vi "target.vi"   [LabVIEW 2020]
uses:
  <vilib>/rvi/interface/RandomDataEmulation/niFpgaRandomDataHandleErrors.vi
  <vilib>/rvi/DataTransferAndStorage/Container/XNode/niFpgaContainer.xnode
  <vilib>/rvi/interface/RandomDataEmulation/nirviRandomDataFpgaReadWriteTemplate.vi
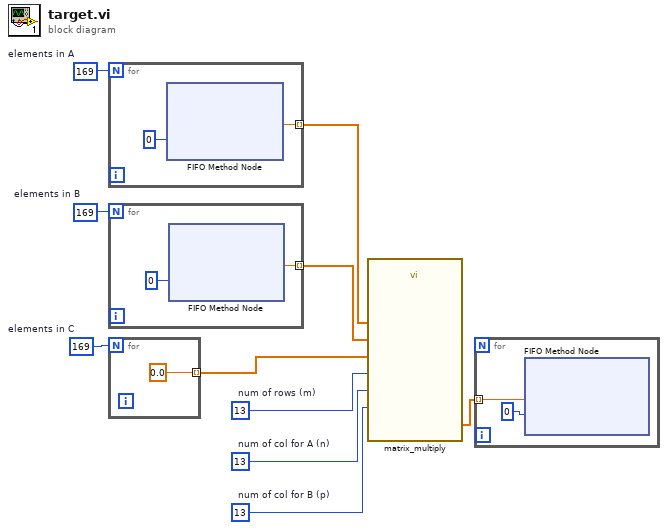
[diagram p0: block diagram]
diagram:
  w2 = 169  # elements in C
  w9 = 169  # elements in B
  w7 = 13  # num of col for B (p)
  w6 = 13  # num of col for A (n)
  w5 = 13  # num of rows (m)
  w10 = 169  # elements in A
  n1 = for {
    N: w10 -> [_]
    tunnel: [w12] -> w4 mode=indexing
    n2 = xnode ("FIFO Method Node")("Timeout"=0) -> ("Element"=w12:sgl)  [unwired: 1 in, 2 out]
  }
  n3 = for {
    N: w9 -> [_]
    tunnel: [w13] -> w3 mode=indexing
    n4 = xnode ("FIFO Method Node")("Timeout"=0) -> ("Element"=w13:sgl)  [unwired: 1 in, 2 out]
  }
  n5 = for {
    N: w2 -> [_]
    tunnel: [sgl 0.0] -> w1 mode=indexing
  }
  n6 = call "matrix_multiply.vi"("p"=w7, "C"=w1, "n"=w6, "m"=w5, "B"=w3, "A"=w4) -> ("C"=w8:sgl[])
  n7 = for {
    tunnel: w8 -> [w17] mode=indexing
    n8 = xnode ("FIFO Method Node")("Element"=w17, "Timeout"=0) -> ()  [unwired: 1 in, 2 out]
  }
